vi "compress_tiff_buffer_example.vi"() -> ()   [LabVIEW 2020]
panel:
  out "dp_status_init":i32
  out "dp_status_prepare":i32
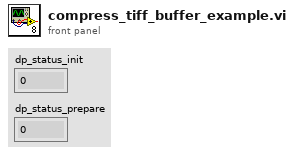
[diagram p1: front panel]
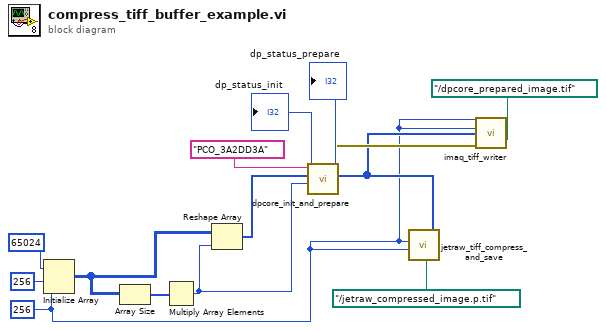
[diagram p0: block diagram]
diagram:
  w1 = 256 ("dimension size")
  n1 = Initialize Array(65024 ("element"), 256 ("dimension size"), w1) -> (w4:i32[][])
  n2 = Array Size(array=w4) -> (size(s)=w5:i32[])
  n3 = Multiply Array Elements(1:w5) -> (0:w2:i32)
  n4 = Reshape Array(w4, w2) -> (w3:i32[])
  n5 = call "dpcore_init_and_prepare.vi"("image_length"=w2, "Image Pixels (U16)"=w3, "identifier"="PCO_3A2DD3A" ("file_path")) -> ("error out"=w11:errorcluster, "dp_status_prepare"=→"dp_status_prepare":i32, "prepared_image_buffer"=w9:u16[], "dp_status_init"=→"dp_status_init":i32)  [unwired: 5 in]
  n6 = call "jetraw_tiff_compress_and_save.vi"("compressed output filename"=path "../jetraw_compressed_image.p.tif" ("name or relative path"), "height"=w1, "width"=w1, "image_buffer"=w9) -> ()  [unwired: 8 in]
  n7 = call "imaq_tiff_writer.vi"("image_width"=w1, "image_height"=w1, "output_buffer in"=w9, "name or relative path"=path "../dpcore_prepared_image.tif", "error in (no error)"=w11) -> ()  [unwired: 11 in]
